vi "主面板.vi"() -> ()   [LabVIEW 2012]
panel:
  in  "关于作者":bool
  in  "刷新":bool
  out "stories":T1(array[cluster])
  out "top_stories":cluster{"字符串 2":string, "二维图片":picture}[](array[cluster])
  out "title with pic":cluster{"字符串 2":string, "二维图片":picture}[](array[cluster])
  in  "WebBrowser":refnum<k7>(container) caption="网页浏览器"
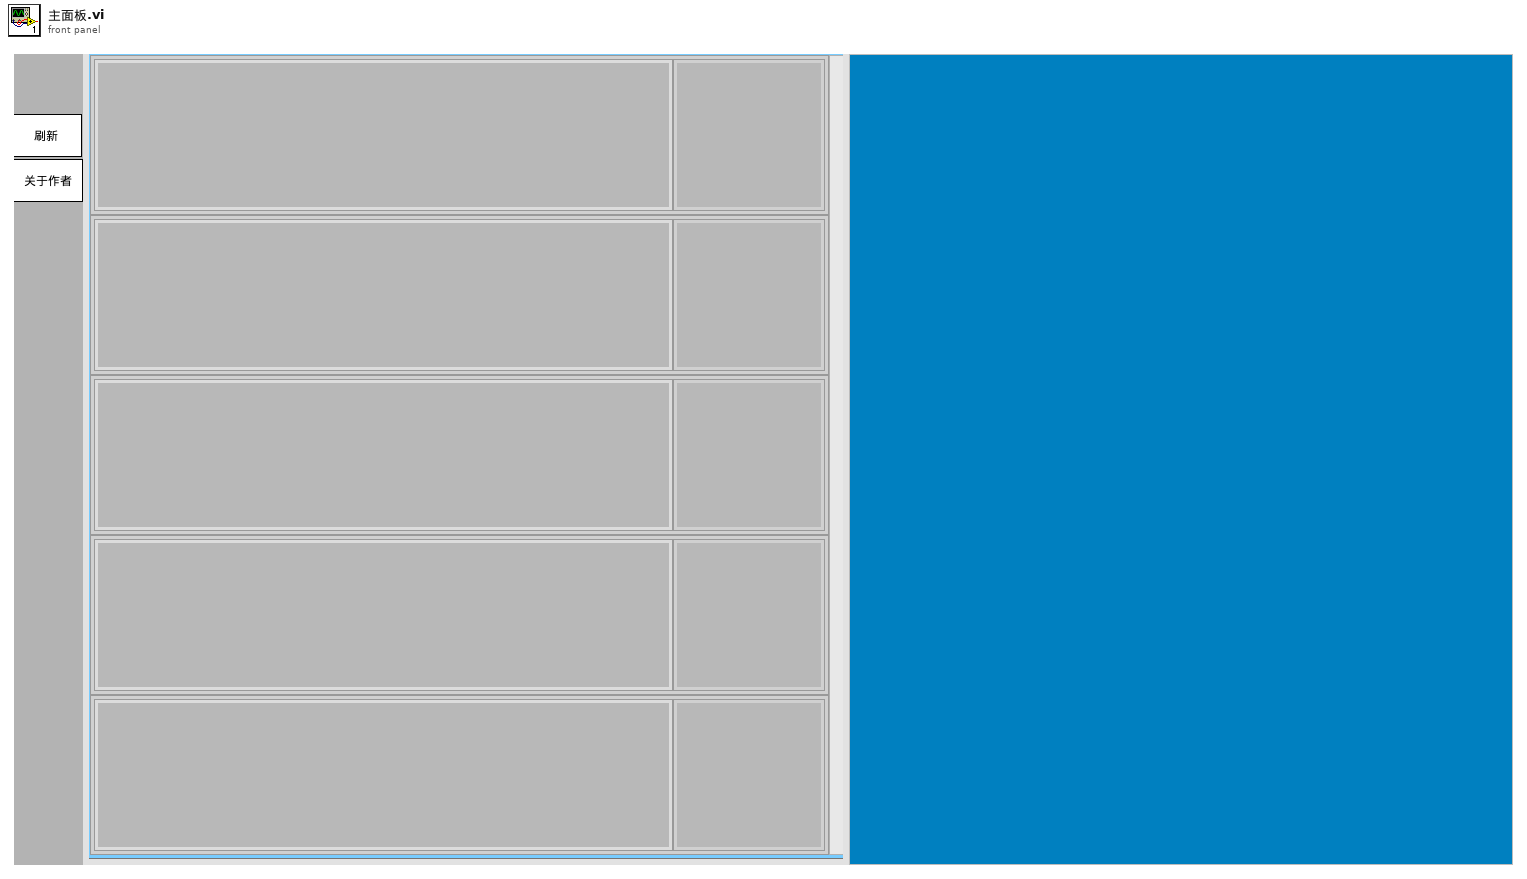
[diagram p1: front panel]
types:
  T1 = cluster{"images":string, "type":i32, "id":i64, "ga_prefix":string, "title":string}[]
  T2 = cluster{"images":string, "type":i32, "id":i64, "ga_prefix":string, "title":string}
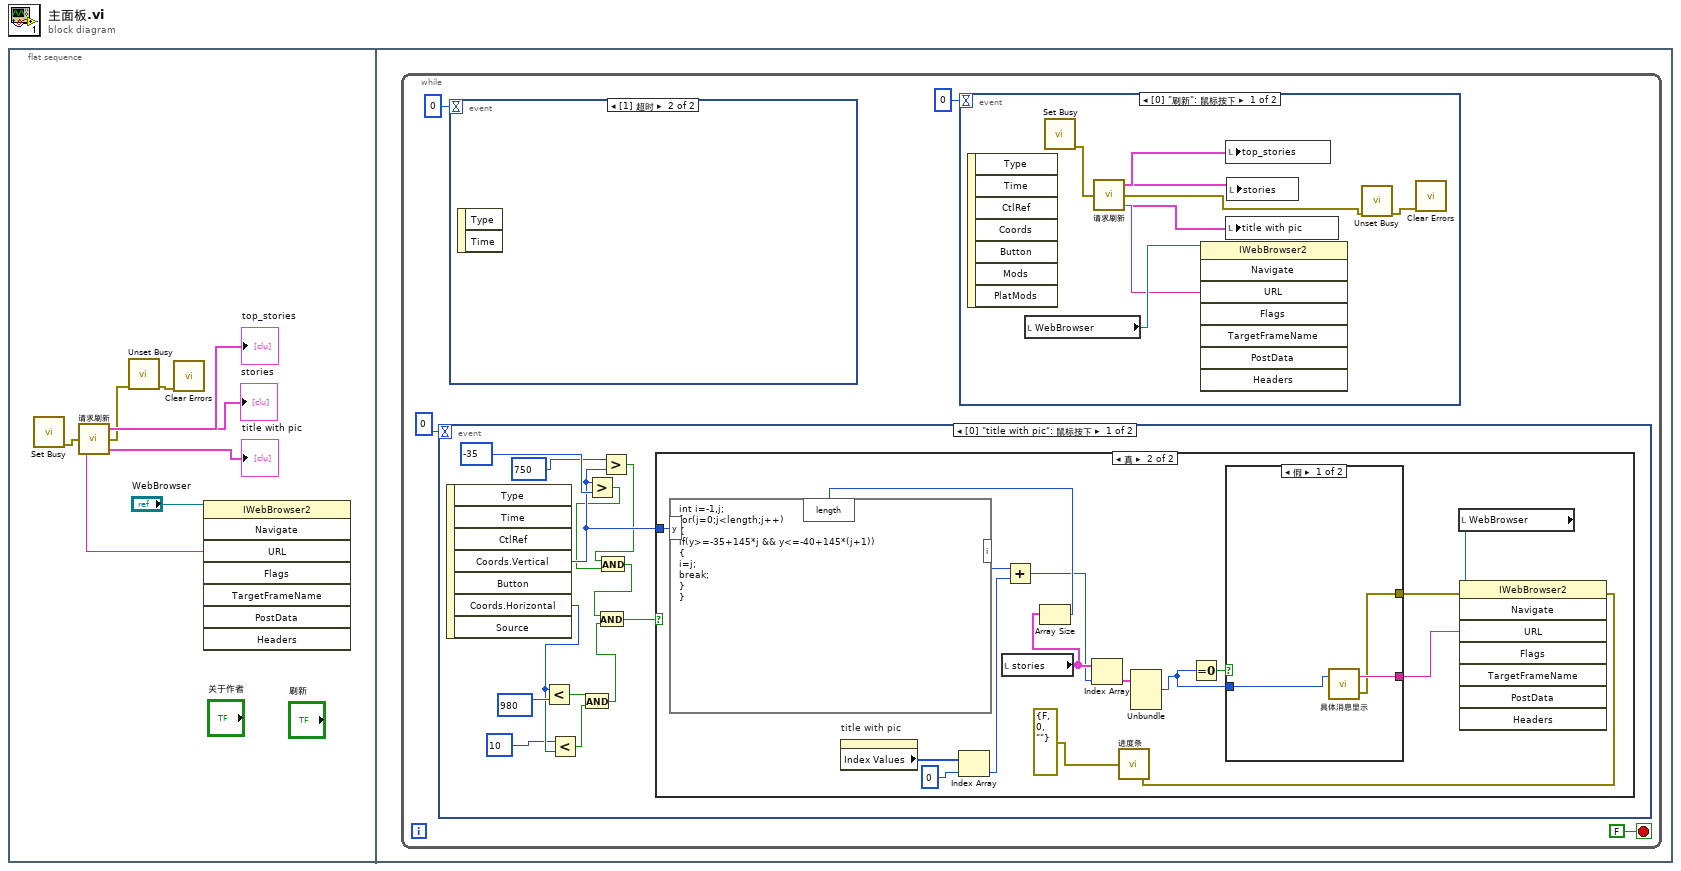
[diagram p0: block diagram]
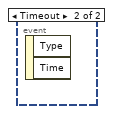
[diagram p2: hidden frame]
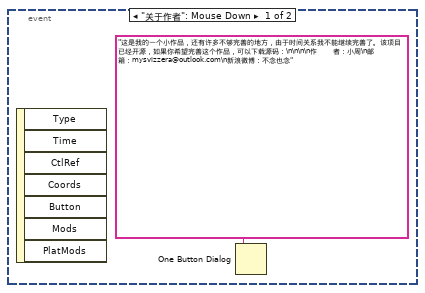
[diagram p3: hidden frame]
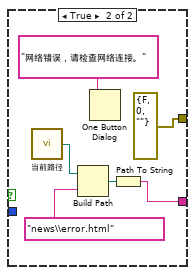
[diagram p5: hidden frame]
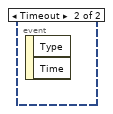
[diagram p6: hidden frame]
diagram:
  n1 = flat-sequence {
    frame #0 {
      n2 = call <vilib>:"Set Busy.vi"() -> ("error out"=w3:errorcluster)  [unwired: 10 in, 1 out]
      n3 = call "请求刷新.vi"("Error Out"=w3) -> ("title with pic"=→"title with pic":cluster{"字符串 2":string, "二维图片":picture}[], "error out"=w1:errorcluster, "stories"=→"stories":T1, "URL"=w4:string, "top_stories"=→"top_stories":cluster{"字符串 2":string, "二维图片":picture}[])
      n4 = call <vilib>:"Unset Busy.vi"("error in (no error)"=w1) -> ("error out"=w2:errorcluster)  [unwired: 10 in]
      n5 = call <vilib>:"Clear Errors.vi"("error in (no error)"=w2) -> ()  [unwired: 6 in, 1 out]
      n6 = invoke class="IWebBrowser2" method="Navigate"(reference="WebBrowser", "URL"=w4) -> ()  [unwired: 6 in, 8 out]
    }
    frame #1 {
      n7 = while {
        stop <- FALSE stop-if-true
        n8 = event shown="[0] \"title with pic\": 鼠标按下" {
          selector: _ -> [_ _]
          dyn-events: _ -> [_ _]
          timeout: 0 -> [_ _]
          event "title with pic": Mouse Down {
            n9 = event-data() -> ("Coords.Vertical"=w31:i32, "Coords.Horizontal"=w26:i32)  [unwired: 1 in, 5 out]
            n10 = Less?(x=w26, y=980) -> (x < y?=w24:bool)
            n11 = Less?(x=10, y=w26) -> (x < y?=w23:bool)
            n12 = And(x=w24, y=w23) -> (x .and. y?=w22:bool)
            n13 = Greater?(x=w31, y=-35) -> (0:w28:bool)
            n14 = Greater?(x=750, y=w31) -> (0:w29:bool)
            n15 = And(x=w29, y=w28) -> (x .and. y?=w27:bool)
            n16 = And(x=w27, y=w22) -> (x .and. y?=w32:bool)
            n17 = case shown="真" w32 {
              tunnel: w31 -> [_ w39]
              frame False {
              }
              frame True {
                n18 = property on="title with pic" class="Arr (严格)"() -> ("Index Values"=w42:u32[])  [unwired: 2 in, 2 out]
                n19 = Index Array(array=w42, index=0) -> (element=w40:u32)
                n20 = local read "stories"() -> (w45:T1)
                n21 = Array Size(array=w45) -> (size(s)=w46:i32)
                n22 = formula code="int i=-1,j;\nfor(j=0;j<length;j++)\n{\nif(y>=-35+145*j && y<=-40+145*(j+1))\n{\ni=j;\nbreak;\n}\n}"("y"=w39, "length"=w46) -> ("i"=w43:i32)
                n23 = Add(x=w43, y=w40) -> (x+y=w38:u32)
                n24 = Index Array(array=w45, index=w38) -> (element=w50:T2)
                n25 = Unbundle(w50) -> ("id"=w47:i64)  [unwired: 4 out]
                n26 = Equal To 0?(x=w47) -> (x = 0?=w48:bool)
                n27 = case shown="假" w48 {
                  tunnel: w47 -> [w53 _]
                  tunnel: [w52 w56] -> w44
                  tunnel: [w51 errorcluster {"status"=FALSE, "code"=0, "source"=""} ("error out")] -> w36
                  frame False {
                    n28 = call "具体消息显示.vi"("ID"=w53) -> ("error out"=w51:errorcluster, "html_url"=w52:string)  [unwired: 1 in]
                  }
                  frame True {
                    n29 = call "当前路径.vi"() -> ("路径"=w57:path)
                    n30 = Build Path(base path=w57, name or relative path="news\\error.html") -> (appended path=w59:path)
                    n31 = One Button Dialog(message="网络错误，请检查网络连接。") -> ()  [unwired: 1 in, 1 out]
                    n32 = Path To String(path=w59) -> (string=w56:string)
                  }
                }
                n33 = local read "WebBrowser"() -> (w49:refnum<k7>)
                n34 = invoke class="IWebBrowser2" method="Navigate"(reference=w49, error in=w36, "URL"=w44) -> (error out=w35:errorcluster)  [unwired: 5 in, 7 out]
                n35 = call "进度条.vi"("error out"=w35, "Error Out"=errorcluster {"status"=FALSE, "code"=0, "source"=""} ("error in (no error)")) -> ()
              }
            }
          }
          event Timeout {
            n36 = event-data() -> ()  [unwired: 1 in, 2 out]
          }
        }
        n37 = event shown="[1] 超时" {
          selector: _ -> [_ _]
          dyn-events: _ -> [_ _]
          timeout: 0 -> [_ _]
          event "关于作者": Mouse Down {
            n38 = event-data() -> ()  [unwired: 1 in, 7 out]
            n39 = One Button Dialog(message="这是我的一个小作品，还有许多不够完善的地方，由于时间关系我不能继续完善了。该项目已经开源，如果你希望完善这个作品，可以下载源码：\n\n\n\n作        者：小周\n邮        箱：mysvizzera@outlook.com\n新浪微博：不念也念") -> ()  [unwired: 1 in, 1 out]
          }
          event Timeout {
            n40 = event-data() -> ()  [unwired: 1 in, 2 out]
          }
        }
        n41 = event shown="[0] \"刷新\": 鼠标按下" {
          selector: _ -> [_ _]
          dyn-events: _ -> [_ _]
          timeout: 0 -> [_ _]
          event "刷新": Mouse Down {
            n42 = event-data() -> ()  [unwired: 1 in, 7 out]
            n43 = local read "WebBrowser"() -> (w20:refnum<k7>)
            n44 = call <vilib>:"Set Busy.vi"() -> ("error out"=w14:errorcluster)  [unwired: 10 in, 1 out]
            n45 = call "请求刷新.vi"("Error Out"=w14) -> ("title with pic"=w16:cluster{"字符串 2":string, "二维图片":picture}[], "error out"=w13:errorcluster, "stories"=w17:T1, "URL"=w19:string, "top_stories"=w18:cluster{"字符串 2":string, "二维图片":picture}[])
            n46 = invoke class="IWebBrowser2" method="Navigate"(reference=w20, "URL"=w19) -> ()  [unwired: 6 in, 8 out]
            n47 = local write "top_stories"(w18) -> ()
            n48 = local write "title with pic"(w16) -> ()
            n49 = local write "stories"(w17) -> ()
            n50 = call <vilib>:"Unset Busy.vi"("error in (no error)"=w13) -> ("error out"=w15:errorcluster)  [unwired: 10 in]
            n51 = call <vilib>:"Clear Errors.vi"("error in (no error)"=w15) -> ()  [unwired: 6 in, 1 out]
          }
          event Timeout {
            n52 = event-data() -> ()  [unwired: 1 in, 2 out]
          }
        }
      }
    }
  }
